vi "Write Fast.vi"(8 "error in (no error)":errorcluster, 9 "Value":variant, 10 "Name":string, 11 "TwinCAT ADS in":refnum<class "TwinCAT ADS.lvclass">) -> (0 "error out":errorcluster, 3 "TwinCAT ADS out":refnum<class "TwinCAT ADS.lvclass">)   [LabVIEW 2018, in "TwinCAT ADS.lvclass"]
uses:
  TwinCAT ADS.lvclass
  TwinCAT.Ads
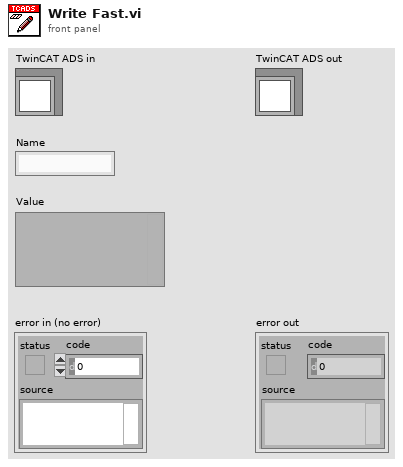
[diagram p1: front panel]
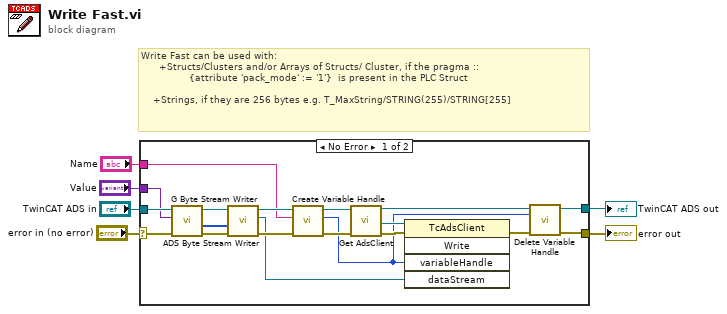
[diagram p0: block diagram]
diagram:
  # "Write Fast can be used with: \n      +Structs/Clusters and/or Arrays of Structs/ Cluster, if the pragma :: \n                {attribute 'pack_mode' := '1'}  is present in the PLC Struct\n\n    +Strings, if they are 256 bytes e.g. T_MaxString/STRING(255)/STRING[255]"
  n1 = case shown="No Error" "error in (no error)" {
    selector: "error in (no error)" -> [w24 w26]
    tunnel: "Value" -> [w23 _]
    tunnel: "TwinCAT ADS in" -> [w25 w27]
    tunnel: [w8 w27] -> w2
    tunnel: "Name" -> [w17 _]
    tunnel: [w9 w26] -> w1
    frame No Error {
      n2 = call-dynamic "G Byte Stream Writer.vi"("error in (no error)"=w24, "Value"=w23, "TwinCAT ADS in"=w25) -> ("error out"=w22:errorcluster, "Byte Stream"=w20:u8[], "TwinCAT ADS out"=w21:refnum<class "TwinCAT ADS.lvclass">)  [unwired: 6 in]
      n3 = call "ADS Byte Stream Writer.vi"("error in (no error)"=w22, "Byte Stream In"=w20, "TwinCAT ADS in"=w21) -> ("error out"=w19:errorcluster, ".NET AdsStream"=w7:refnum<k24>, "TwinCAT ADS out"=w18:refnum<class "TwinCAT ADS.lvclass">)  [unwired: 5 in, 1 out]
      n4 = call-dynamic "Create Variable Handle.vi"("error in (no error)"=w19, "Name"=w17, "TwinCAT ADS in"=w18) -> ("error out"=w16:errorcluster, "Handle"=w10:i32, "TwinCAT ADS out"=w15:refnum<class "TwinCAT ADS.lvclass">)  [unwired: 6 in]
      n5 = call-dynamic "Get AdsClient.vi"("error in (no error)"=w16, "TwinCAT ADS in"=w15) -> ("error out"=w14:errorcluster, ".NET TcAdsClient refnum"=w13:refnum<k24>, "TwinCAT ADS out"=w11:refnum<class "TwinCAT ADS.lvclass">)  [unwired: 7 in]
      n6 = invoke class="TcAdsClient" method="Write"(reference=w13, error in=w14, "variableHandle"=w10, "dataStream"=w7) -> (error out=w12:errorcluster)  [unwired: 1 in, 4 out]
      n7 = call-dynamic "Delete Variable Handle.vi"("error in (no error)"=w12, "Handle"=w10, "TwinCAT ADS in"=w11) -> ("error out"=w9:errorcluster, "TwinCAT ADS out"=w8:refnum<class "TwinCAT ADS.lvclass">)  [unwired: 7 in]
    }
    frame Error {
    }
  }
  "error out" <- w1
  "TwinCAT ADS out" <- w2
